vi "Add.vi"(8 "error in (no error)":errorcluster, 9 "Alias":string, 10 "Topic":string, 11 "DICT in":refnum<class "DICT.lvclass">) -> (0 "error out":errorcluster, 3 "DICT out":refnum<class "DICT.lvclass">)   [LabVIEW 2017, in "DICT.lvclass"]
uses:
  DICT.lvclass
  DICT.lvclass/DICT.ctl
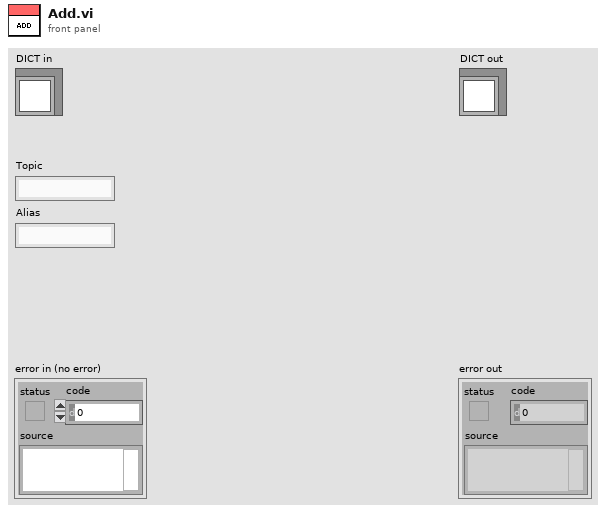
[diagram p1: front panel]
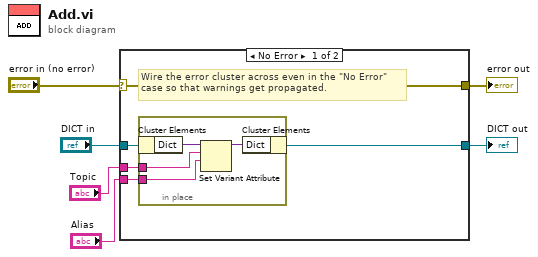
[diagram p0: block diagram]
diagram:
  n1 = case shown="No Error" "error in (no error)" {
    selector: "error in (no error)" -> [w11 w17]
    tunnel: [w11 w17] -> w5
    tunnel: [w9 w16] -> w3
    tunnel: "DICT in" -> [w10 w16]
    tunnel: "Topic" -> [w8 _]
    tunnel: "Alias" -> [w7 _]
    frame No Error {
      # "Wire the error cluster across even in the \"No Error\"\ncase so that warnings get propagated."
      n2 = in-place {
        in-place-border: w8 -> [w13]
        in-place-border: w7 -> [w12]
        n3 = in-place-cluster #1(w10) -> ("Dict"=w15:variant)
        n4 = Set Variant Attribute(Variant=w15, name=w13, value=w12) -> (Variant out=w14:variant)  [unwired: 1 in, 2 out]
        n5 = in-place-cluster #1("Dict"=w14) -> (w9:refnum<class "DICT.lvclass">)
      }
    }
    frame Error {
    }
  }
  "error out" <- w5
  "DICT out" <- w3
